vi "Auton_S1_Left_Scale_Left_Switch_2Cube.vi"   [LabVIEW 2017]
uses:
  <vilib>/Rock Robotics/WPI/Utilities/WPI_GetSetVariantRefNum.vi
  Robot Global Data.vi
  <vilib>/Rock Robotics/WPI/RobotDrive/WPI_RobotDriveArcadeDrive_Standard(NoSaturation).vi
types:
  T1 = typedef "WPI_RobotDriveDevRef.ctl" = cluster{"DevStatus":errorcluster, "Motors[]":T2[], "Square Inputs":bool, "Max Output":dbl}
  T2 = typedef "WPI_MotorControlDeviceRef.ctl" = cluster{"DeviceStatus":errorcluster, "Type":T3, "PWM":cluster{"PWM Channel":T4, "DeadBand":T5}, "CAN":cluster{"Device Number":u8, "SetOutput VI Ref":variant, "GetOutput VI Ref":variant, "Enable VI Ref":variant, "Disable VI Ref":variant, "Data":variant}, "Invert":bool, "DIO PWM":cluster{"PWM \"Enable\" Channel":T4, "DIOChannel":T6, "PWM Rate":dbl}}
  T3 = typedef "WPI_MotorControlType.ctl" = enum16{"PWM", "CAN", "DIO PWM"}
  T4 = typedef "FPGA_DIOPWMChannel.ctl" = enum8{"PWM 0", "PWM 1", "PWM 2", "PWM 3", "PWM 4", "PWM 5", "PWM 6", "PWM 7", "PWM 8", "PWM 9", "PWM MXP 0", "PWM MXP 1", "PWM MXP 2", "PWM MXP 3", "PWM MXP 4", "PWM MXP 5", "PWM MXP 6", "PWM MXP 7", "PWM MXP 8", "PWM MXP 9", "Invalid"}
  T5 = typedef "WPI_PWMDeadband.ctl" = cluster{"Name":string, "maxPositivePwm":i32, "minPositivePwm":i32, "centerPwm":i32, "maxNegativePwm":i32, "minNegativePwm":i32, "angularRange":u16}
  T6 = typedef "FPGA_DIOChannel.ctl" = enum8{"DIO 0", "DIO 1", "DIO 2", "DIO 3", "DIO 4", "DIO 5", "DIO 6", "DIO 7", "DIO 8", "DIO 9", "DIO MXP 0", "DIO MXP 1", "DIO MXP 2", "DIO MXP 3", "DIO MXP 4", "DIO MXP 5", "DIO MXP 6", "DIO MXP 7", "DIO MXP 8", "DIO MXP 9", "DIO MXP 10", "DIO MXP 11", "DIO MXP 12", "DIO MXP 13", "DIO MXP 14", "DIO MXP 15", "SPI Port CS1", "SPI Port CS2", "SPI Port CS3", "SPI Port MISO", "SPI Port MOSI", "Invalid"}
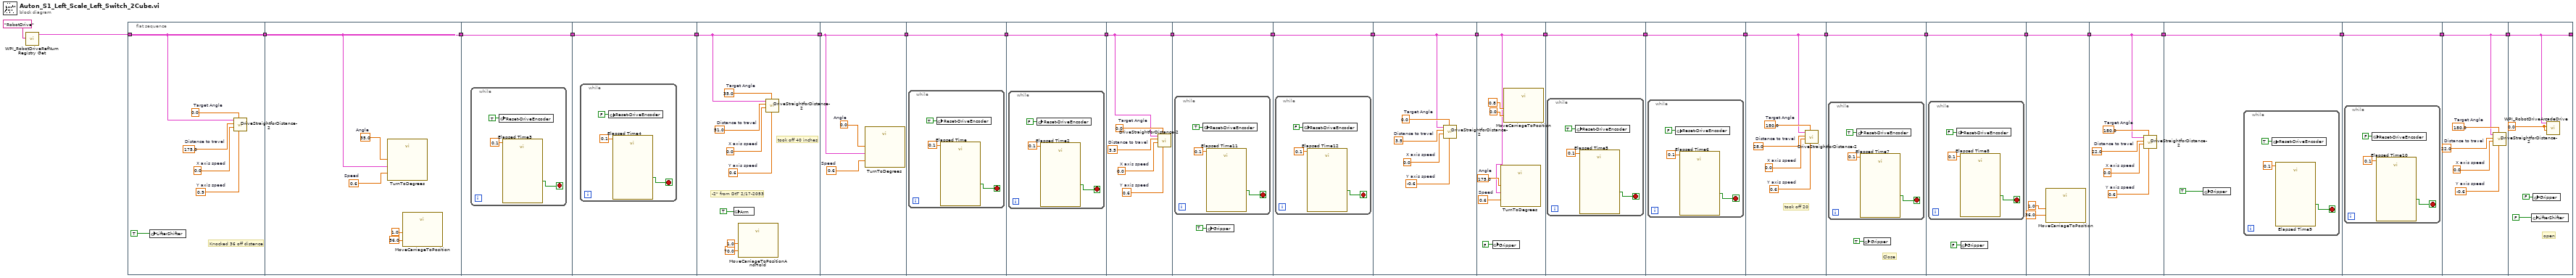
[diagram p0: block diagram]
diagram:
  n1 = call <vilib>:"WPI_RobotDriveRefNum Registry Get.vi"("refnum name"="RobotDrive") -> ("RobotDriveDevRef"=w22:T1)  [unwired: 9 in, 1 out]
  n2 = flat-sequence {
    tunnel: [w31] -> w3
    tunnel: w22 -> [w31]
    tunnel: [w35] -> w25
    tunnel: w3 -> [w35]
    tunnel: w25 -> [w37]
    tunnel: [w37] -> w24
    tunnel: [w41] -> w21
    tunnel: w24 -> [w41]
    tunnel: w21 -> [w48]
    tunnel: [w48] -> w9
    tunnel: w9 -> [w53]
    tunnel: [w53] -> w8
    tunnel: w8 -> [w56]
    tunnel: [w56] -> w20
    tunnel: w20 -> [w60]
    tunnel: [w60] -> w19
    tunnel: w19 -> [w64]
    tunnel: [w64] -> w7
    tunnel: w7 -> [w70]
    tunnel: [w70] -> w5
    tunnel: w5 -> [w74]
    tunnel: [w74] -> w4
    tunnel: w4 -> [w78]
    tunnel: [w78] -> w6
    tunnel: w6 -> [w84]
    tunnel: [w84] -> w18
    tunnel: w18 -> [w89]
    tunnel: [w89] -> w17
    tunnel: w17 -> [w93]
    tunnel: [w93] -> w16
    tunnel: w16 -> [w97]
    tunnel: [w97] -> w15
    tunnel: w15 -> [w103]
    tunnel: [w103] -> w14
    tunnel: w14 -> [w108]
    tunnel: [w108] -> w2
    tunnel: w2 -> [w114]
    tunnel: [w114] -> w1
    tunnel: w1 -> [w115]
    tunnel: [w115] -> w13
    tunnel: [w121] -> w12
    tunnel: w13 -> [w121]
    tunnel: w12 -> [w125]
    tunnel: [w125] -> w11
    tunnel: w11 -> [w129]
    tunnel: [w129] -> w10
    tunnel: [w136] -> _
    tunnel: w10 -> [w136]
    frame #0 {
      w27 = 0.0  # Target Angle
      w28 = 0.9  # Y axis speed
      w29 = 0.0  # X axis speed
      w30 = 175.0  # Distance to travel
      # "Knocked 36 off distence"
      n3 = global write "Robot Global Data.vi" "LifterShifter"(TRUE ("Reset-DriveEncoder")) -> ()
      n4 = call "DriveStraightforDistance-2.vi"("Y axis speed"=w28, "Target Angle"=w27, "X axis speed"=w29, "Distance to travel"=w30, "RobotDriveDevRef"=w31) -> ()  [unwired: 7 in]
    }
    frame #1 {
      w34 = 35.0  # Angle
      w36 = 0.6  # Speed
      n5 = call "TurnToDegrees.vi"("Speed"=w36, "RobotDriveDevRef"=w35, "Angle"=w34) -> ()  [unwired: 9 in]
      n6 = call "MoveCarriageToPosition.vi"("Lift Speed"=1.0, "Target Height"=36.0) -> ()  [unwired: 10 in]
    }
    frame #2 {
      n7 = while {
        stop <- w40 stop-if-true
        n8 = global write "Robot Global Data.vi" "Reset-DriveEncoder"(TRUE ("Reset-DriveEncoder")) -> ()
        n9 = call "Elapsed Time3"("Time Target (s)"=0.1) -> ("Time has Elapsed"=w40:bool)  [unwired: 11 in, 7 out]
      }
    }
    frame #3 {
      n10 = while {
        stop <- w44 stop-if-true
        n11 = global write "Robot Global Data.vi" "Reset-DriveEncoder"(FALSE ("Reset-DriveEncoder")) -> ()
        n12 = call "Elapsed Time4"("Time Target (s)"=0.1) -> ("Time has Elapsed"=w44:bool)  [unwired: 11 in, 7 out]
      }
    }
    frame #4 {
      w49 = 35.0  # Target Angle
      w50 = 0.6  # Y axis speed
      w51 = 0.0  # X axis speed
      w52 = 51.0  # Distance to travel
      # "took off 40 inches"
      # "-2\" from DtT 2/17-2053"
      n13 = global write "Robot Global Data.vi" "Arm"(TRUE ("Gripper")) -> ()
      n14 = call "MoveCarriageToPositionAndHold.vi"("Lift Speed"=1.0, "Target Height"=70.0) -> ()  [unwired: 10 in]
      n15 = call "DriveStraightforDistance-2.vi"("Y axis speed"=w50, "Target Angle"=w49, "X axis speed"=w51, "Distance to travel"=w52, "RobotDriveDevRef"=w48) -> ()  [unwired: 7 in]
    }
    frame #5 {
      w54 = 0.0  # Angle
      w55 = 0.6  # Speed
      n16 = call "TurnToDegrees.vi"("Speed"=w55, "RobotDriveDevRef"=w53, "Angle"=w54) -> ()  [unwired: 9 in]
    }
    frame #6 {
      n17 = while {
        stop <- w59 stop-if-true
        n18 = global write "Robot Global Data.vi" "Reset-DriveEncoder"(TRUE ("Reset-DriveEncoder")) -> ()
        n19 = call "Elapsed Time"("Time Target (s)"=0.1) -> ("Time has Elapsed"=w59:bool)  [unwired: 11 in, 7 out]
      }
    }
    frame #7 {
      n20 = while {
        stop <- w63 stop-if-true
        n21 = global write "Robot Global Data.vi" "Reset-DriveEncoder"(FALSE ("Reset-DriveEncoder")) -> ()
        n22 = call "Elapsed Time2"("Time Target (s)"=0.1) -> ("Time has Elapsed"=w63:bool)  [unwired: 11 in, 7 out]
      }
    }
    frame #8 {
      w65 = 0.0  # Target Angle
      w66 = 0.6  # Y axis speed
      w67 = 0.0  # X axis speed
      w68 = 3.5  # Distance to travel
      n23 = call "DriveStraightforDistance-2.vi"("Y axis speed"=w66, "Target Angle"=w65, "X axis speed"=w67, "Distance to travel"=w68, "RobotDriveDevRef"=w64) -> ()  [unwired: 7 in]
    }
    frame #9 {
      n24 = while {
        stop <- w73 stop-if-true
        n25 = global write "Robot Global Data.vi" "Reset-DriveEncoder"(TRUE ("Reset-DriveEncoder")) -> ()
        n26 = call "Elapsed Time11"("Time Target (s)"=0.1) -> ("Time has Elapsed"=w73:bool)  [unwired: 11 in, 7 out]
      }
      n27 = global write "Robot Global Data.vi" "Gripper"(TRUE ("Gripper")) -> ()
    }
    frame #10 {
      n28 = while {
        stop <- w77 stop-if-true
        n29 = global write "Robot Global Data.vi" "Reset-DriveEncoder"(FALSE ("Reset-DriveEncoder")) -> ()
        n30 = call "Elapsed Time12"("Time Target (s)"=0.1) -> ("Time has Elapsed"=w77:bool)  [unwired: 11 in, 7 out]
      }
    }
    frame #11 {
      w79 = 0.0  # Target Angle
      w80 = -0.6  # Y axis speed
      w81 = 0.0  # X axis speed
      w82 = 3.5  # Distance to travel
      n31 = call "DriveStraightforDistance-2.vi"("Y axis speed"=w80, "Target Angle"=w79, "X axis speed"=w81, "Distance to travel"=w82, "RobotDriveDevRef"=w78) -> ()  [unwired: 7 in]
    }
    frame #12 {
      w85 = 175.0  # Angle
      w86 = 0.6  # Speed
      n32 = global write "Robot Global Data.vi" "Gripper"(FALSE ("Gripper")) -> ()
      n33 = call "TurnToDegrees.vi"("Speed"=w86, "RobotDriveDevRef"=w84, "Angle"=w85) -> ()  [unwired: 9 in]
      n34 = call "MoveCarriageToPosition.vi"("Lift Speed"=0.8, "Target Height"=0.0) -> ()  [unwired: 10 in]
    }
    frame #13 {
      n35 = while {
        stop <- w92 stop-if-true
        n36 = global write "Robot Global Data.vi" "Reset-DriveEncoder"(TRUE ("Reset-DriveEncoder")) -> ()
        n37 = call "Elapsed Time5"("Time Target (s)"=0.1) -> ("Time has Elapsed"=w92:bool)  [unwired: 11 in, 7 out]
      }
    }
    frame #14 {
      n38 = while {
        stop <- w96 stop-if-true
        n39 = global write "Robot Global Data.vi" "Reset-DriveEncoder"(FALSE ("Reset-DriveEncoder")) -> ()
        n40 = call "Elapsed Time6"("Time Target (s)"=0.1) -> ("Time has Elapsed"=w96:bool)  [unwired: 11 in, 7 out]
      }
    }
    frame #15 {
      w98 = 180.0  # Target Angle
      w99 = 0.6  # Y axis speed
      w100 = 0.0  # X axis speed
      w101 = 28.0  # Distance to travel
      # "took off 20"
      n41 = call "DriveStraightforDistance-2.vi"("Y axis speed"=w99, "Target Angle"=w98, "X axis speed"=w100, "Distance to travel"=w101, "RobotDriveDevRef"=w97) -> ()  [unwired: 7 in]
    }
    frame #16 {
      # "Close"
      n42 = while {
        stop <- w106 stop-if-true
        n43 = global write "Robot Global Data.vi" "Reset-DriveEncoder"(TRUE ("Reset-DriveEncoder")) -> ()
        n44 = call "Elapsed Time7"("Time Target (s)"=0.1) -> ("Time has Elapsed"=w106:bool)  [unwired: 11 in, 7 out]
      }
      n45 = global write "Robot Global Data.vi" "Gripper"(TRUE ("Gripper")) -> ()
    }
    frame #17 {
      n46 = while {
        stop <- w111 stop-if-true
        n47 = global write "Robot Global Data.vi" "Reset-DriveEncoder"(FALSE ("Reset-DriveEncoder")) -> ()
        n48 = call "Elapsed Time8"("Time Target (s)"=0.1) -> ("Time has Elapsed"=w111:bool)  [unwired: 11 in, 7 out]
      }
      n49 = global write "Robot Global Data.vi" "Gripper"(FALSE ("Gripper")) -> ()
    }
    frame #18 {
      n50 = call "MoveCarriageToPosition.vi"("Lift Speed"=1.0, "Target Height"=36.0) -> ()  [unwired: 10 in]
    }
    frame #19 {
      w116 = 180.0  # Target Angle
      w117 = 0.6  # Y axis speed
      w118 = 0.0  # X axis speed
      w119 = 22.0  # Distance to travel
      n51 = call "DriveStraightforDistance-2.vi"("Y axis speed"=w117, "Target Angle"=w116, "X axis speed"=w118, "Distance to travel"=w119, "RobotDriveDevRef"=w115) -> ()  [unwired: 7 in]
    }
    frame #20 {
      n52 = global write "Robot Global Data.vi" "Gripper"(TRUE ("Reset-DriveEncoder")) -> ()
      n53 = while {
        stop <- w124 stop-if-true
        n54 = global write "Robot Global Data.vi" "Reset-DriveEncoder"(TRUE ("Reset-DriveEncoder")) -> ()
        n55 = call "Elapsed Time9"("Time Target (s)"=0.1) -> ("Time has Elapsed"=w124:bool)  [unwired: 11 in, 7 out]
      }
    }
    frame #21 {
      n56 = while {
        stop <- w128 stop-if-true
        n57 = global write "Robot Global Data.vi" "Reset-DriveEncoder"(FALSE ("Reset-DriveEncoder")) -> ()
        n58 = call "Elapsed Time10"("Time Target (s)"=0.1) -> ("Time has Elapsed"=w128:bool)  [unwired: 11 in, 7 out]
      }
    }
    frame #22 {
      w130 = 180.0  # Target Angle
      w131 = -0.6  # Y axis speed
      w132 = 0.0  # X axis speed
      w133 = 22.0  # Distance to travel
      n59 = call "DriveStraightforDistance-2.vi"("Y axis speed"=w131, "Target Angle"=w130, "X axis speed"=w132, "Distance to travel"=w133, "RobotDriveDevRef"=w129) -> ()  [unwired: 7 in]
    }
    frame #23 {
      w137 = 0.0 ("X axis value")
      # "open"
      n60 = global write "Robot Global Data.vi" "LifterShifter"(FALSE ("Reset-DriveEncoder")) -> ()
      n61 = global write "Robot Global Data.vi" "Gripper"(FALSE ("Gripper")) -> ()
      n62 = call-poly <vilib>:"WPI_RobotDriveArcadeDrive.vi"("Y axis value"=w137, "X axis value"=w137, "RobotDriveDevRef"=w136) -> ()  [unwired: 6 in, 3 out]
    }
  }
